vi "open automation reference.vi"(8 "error in (no error)":errorcluster, 11 "BMC in":refnum<class "BMC.lvclass">) -> (0 "error out":errorcluster, 3 "BMC out":refnum<class "BMC.lvclass">)   [LabVIEW 2012, in "BMC.lvclass"]
uses:
  BMC.lvclass
  BMC.lvclass/BMC.ctl
panel:
  out "Automation Refnum":refnum<k7>
  in  "CIUsbLib.hostdrv":refnum<k7>
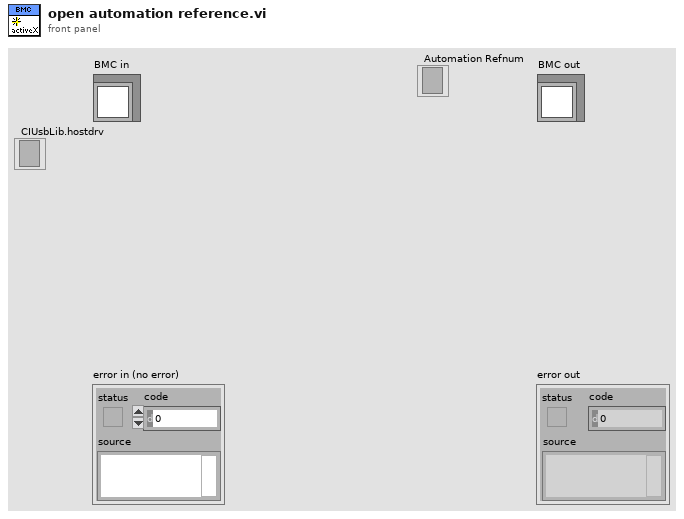
[diagram p1: front panel]
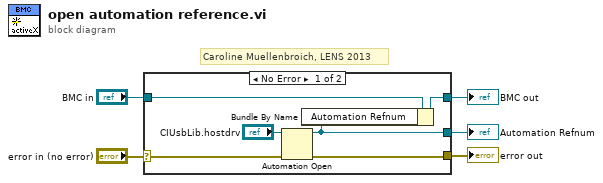
[diagram p0: block diagram]
diagram:
  # "Caroline Muellenbroich, LENS 2013"
  n1 = case shown="No Error" "error in (no error)" {
    selector: "error in (no error)" -> [w11 w13]
    tunnel: [w7 w13] -> w4
    tunnel: "BMC in" -> [w9 w12]
    tunnel: [w10 w12] -> w2
    tunnel: [w6 _] -> w1
    frame No Error {
      n2 = Automation Open(error in (no error)=w11, Automation Refnum="CIUsbLib.hostdrv") -> (Automation Refnum=w6:refnum<k7>, error out=w7:errorcluster)  [unwired: 2 out]
      n3 = Bundle By Name(cluster=w9, "Automation Refnum"=w6) -> (w10:refnum<class "BMC.lvclass">)
    }
    frame Error {
    }
  }
  "error out" <- w4
  "BMC out" <- w2
  "Automation Refnum" <- w1
